vi "DIAG_STM Set Meta Data (TCP Clst).vi"(7 "Meta data":T2[](array[typedef]), 8 "error in":errorcluster, 11 "Connection Info In":T1) -> (0 "error out":errorcluster, 3 "Connection Info Out":T1)   [LabVIEW 2013, in "Diagnostics Addon Engine.lvlib"]
doc: "Assigns the meta data cluster associated with this STM session."
uses:
  Diagnostics Addon Engine.lvlib
  stm_TCP Connection Info.ctl
  _SubVIs/stm_MetaDataElement.ctl
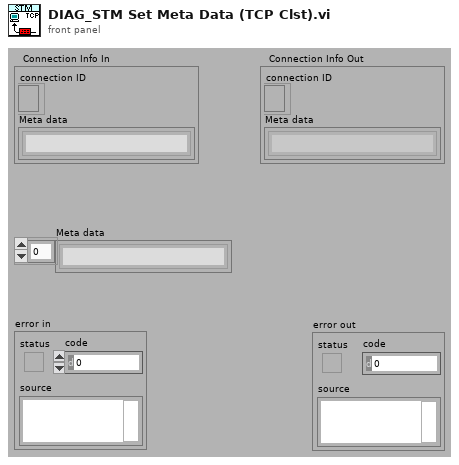
[diagram p1: front panel]
types:
  T1 = typedef "Diagnostics Addon Engine.lvlib/stm_TCP Connection Info.ctl" = cluster{"connection ID":refnum<k5>, "Meta data":T2[]}
  T2 = typedef "Diagnostics Addon Engine.lvlib/stm_MetaDataElement.ctl" = string
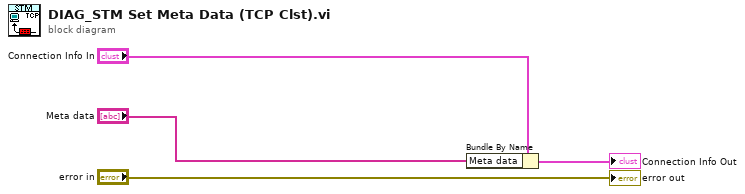
[diagram p0: block diagram]
diagram:
  n1 = Bundle By Name(cluster="Connection Info In", "Meta data"="Meta data") -> (→"Connection Info Out":T1)
  "error out" <- "error in"
